vi "Inverse Square Root 1.vi"() -> ()   [LabVIEW 2022 SP3, in "Benchmark.lvlib"]
uses:
  Benchmark.lvlib
  3ca7c682-72f9-471a-94d6-f3f625e42330.vi
  717569c3-c8f8-4444-b08c-2f89a2934aa8.vi
  <vilib>/Utility/High Resolution Relative Seconds.vi
  <vilib>/Analysis/NI_AALBase.lvlib
panel:
  out "Std Dev":dbl format="%.1p"
  out "Mean":dbl format="%.1p"
  out "Histogram Graph":T1(graph)
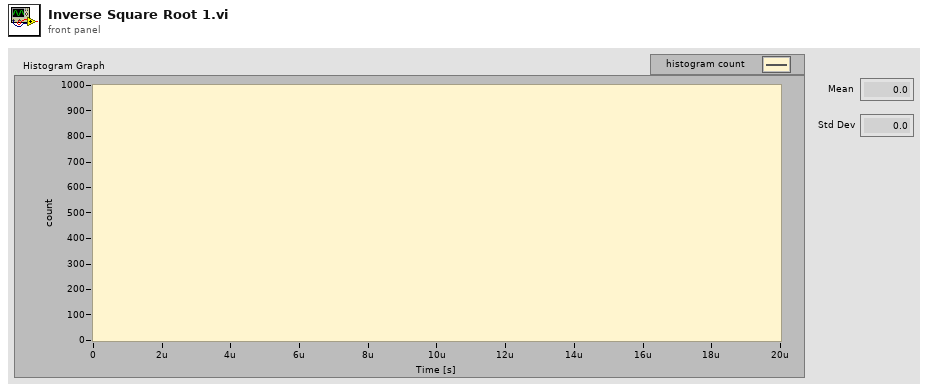
[diagram p1: front panel]
types:
  T1 = cluster{"X Values":dbl[], "Histogram: h(x)":i32[]}
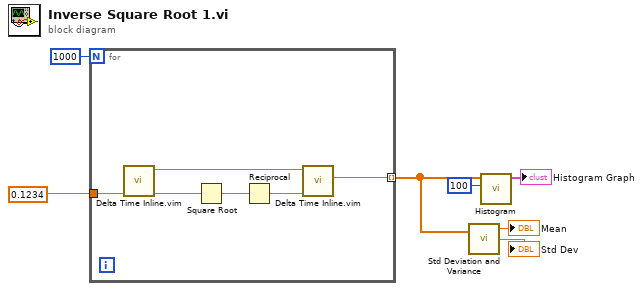
[diagram p0: block diagram]
diagram:
  n1 = for {
    N: 1000 -> [_]
    tunnel: [w13] -> w4 mode=indexing
    tunnel: 0.1234 -> [w10]
    n2 = call "Delta Time Inline.vim"("value in"=w10) -> ("value out"=w11:dbl, "Relative Seconds out [s]"=w12:dbl)  [unwired: 8 in, 1 out]
    n3 = Square Root(x=w11) -> (sqrt(x)=w9:dbl)
    n4 = Reciprocal(x=w9) -> (1/x=w8:dbl)
    n5 = call "Delta Time Inline.vim"("value in"=w8, "Relative Seconds in [s]"=w12) -> ("Delta Time [s]"=w13:dbl)  [unwired: 7 in, 2 out]
  }
  n6 = call <vilib>:"Std Deviation and Variance.vi"("X"=w4) -> ("mean"=→"Mean":dbl, "standard deviation"=→"Std Dev":dbl)  [unwired: 1 in, 1 out]
  n7 = call <vilib>:"Histogram.vi"("intervals"=100, "X"=w4) -> ("Histogram Graph"=→"Histogram Graph":T1)  [unwired: 6 in, 3 out]
